vi "RSNRPZ Get Scope Measurements Offset Time.vi"(8 "error in (no error)":errorcluster, 10 "Channel (1)":i32=1, 11 "VISA session":refnum<visa-resource-name> caption="VISA resource name") -> (0 "error out":errorcluster, 1 "Offset Time":dbl format="%^.3e", 3 "dup VISA session":refnum<visa-resource-name> caption="VISA resource name")   [LabVIEW 2010]
doc: "This VI queries offset time used to set the start point of analysing the current trace for the pulse parameters.\n\nNote:\n1) This VI is only available for NRP-Z81.\n\nRemote-control command(s):\nSENSe:TRACe:MEAS:OFFS:TIME?"
uses:
  rsnrpz_32.dll
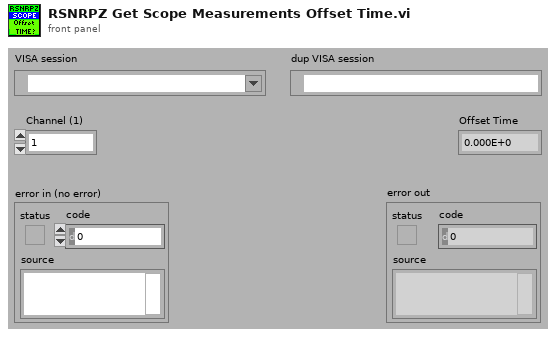
[diagram p1: front panel]
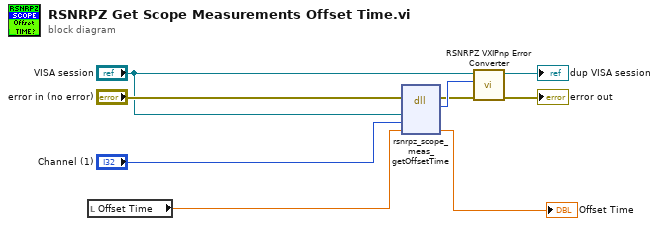
[diagram p0: block diagram]
diagram:
  n1 = local read "Offset Time"() -> (w7:dbl)
  n2 = dll-call lib="rsnrpz_32.dll" fn="rsnrpz_scope_meas_getOffsetTime"(error in="error in (no error)", "Instrument Handle"="VISA session", "Channel"="Channel (1)", "Offset Time"=w7) -> (error out=w5:errorcluster, "Status"=w9:i32, "Offset Time"=→"Offset Time":dbl)  [unwired: 4 in, 1 out]
  n3 = call <instrlib>:"RSNRPZ VXIPnp Error Converter.vi"("error in"=w5, "VXIPnp error code"=w9, "VISA session"="VISA session") -> ("error out"=→"error out":errorcluster, "dup VISA session"=→"dup VISA session":refnum<visa-resource-name>)  [unwired: 7 in]
